vi "MotorOnMain.vi"() -> ()   [LabVIEW 2017]
uses:
  <vilib>/myRIO/Instrument Drivers/Utilities/Utilities.lvlib
panel:
  in  "stop":bool
  out "Error In 2":errorcluster
  in  "Power (%)":dbl
  in  "(Antihorario) Direction (Horario)":bool
  in  "Error In":errorcluster
  in  "Enum":enum16{"MotorB", "MotorA"}(ring)
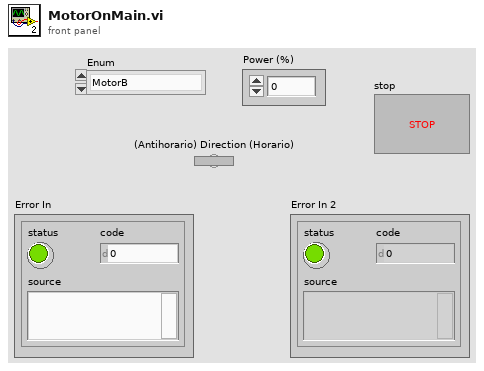
[diagram p1: front panel]
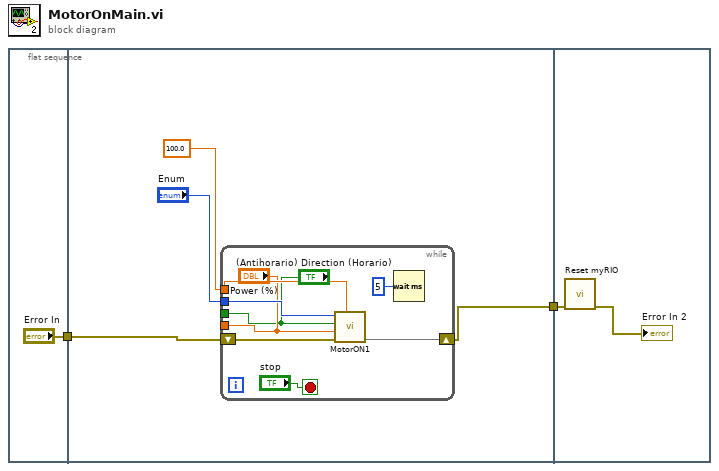
[diagram p0: block diagram]
diagram:
  n1 = flat-sequence {
    tunnel: ["Error In"] -> w1
    tunnel: [w5] -> w2
    tunnel: w1 -> [w4]
    tunnel: w2 -> [w16]
    frame #0 {
    }
    frame #1 {
      n2 = while {
        tunnel: "Enum" -> [w15]
        tunnel: ["(Antihorario) Direction (Horario)"] -> _
        tunnel: ["Power (%)"] -> _
        tunnel: 100.0 ("y") -> [w13]
        shift-right: [w12] -> w5
        shift-left: w4 -> [w14]
        stop <- "stop" stop-if-true
        n3 = call "MotorON1.vi"(7:w13, 8:w14, 9:"Power (%)", 10:"(Antihorario) Direction (Horario)", 11:w15) -> (0:w12)  [unwired: 6 in]
        n4 = Wait (ms)(milliseconds to wait=u32 5) -> ()  [unwired: 1 out]
      }
    }
    frame #2 {
      n5 = call <vilib>:"Reset myRIO.vi"("error in (no error)"=w16) -> ("error out"=→"Error In 2":errorcluster)  [unwired: 10 in]
    }
  }
